vi "Two_neuron_oscillator.vi"() -> ()   [LabVIEW 2016]
uses:
  <vilib>/measure/NI_MABase.lvlib
panel:
  in  "frequency":dbl=0.625 format="%#_13g"
  out "W":T1(graph)
  in  "Modulation":dbl[](array[numeric])=[1.0, 1.0, 1.0, -1.0, 1.0]
  in  "Simulation delay":u32=10
  out "Neurons":T2(graph)
  out "Viewer":T3={"NoPre"=[0, 2, 2], "Pre IDs"=[0, 1, 2, 1, 2], "W"=[1.0, 1.0, 1.0, -1.0, 1.0], "Current"=[1.0, 0.0, 0.0]}
  in  "stop":bool
  in  "Network AER Vectors":T3={"NoPre"=[0, 2, 2], "Pre IDs"=[0, 1, 2, 1, 2], "W"=[1.0, 1.0, 1.0, -1.0, 1.0], "Current"=[1.0, 0.0, 0.0]}
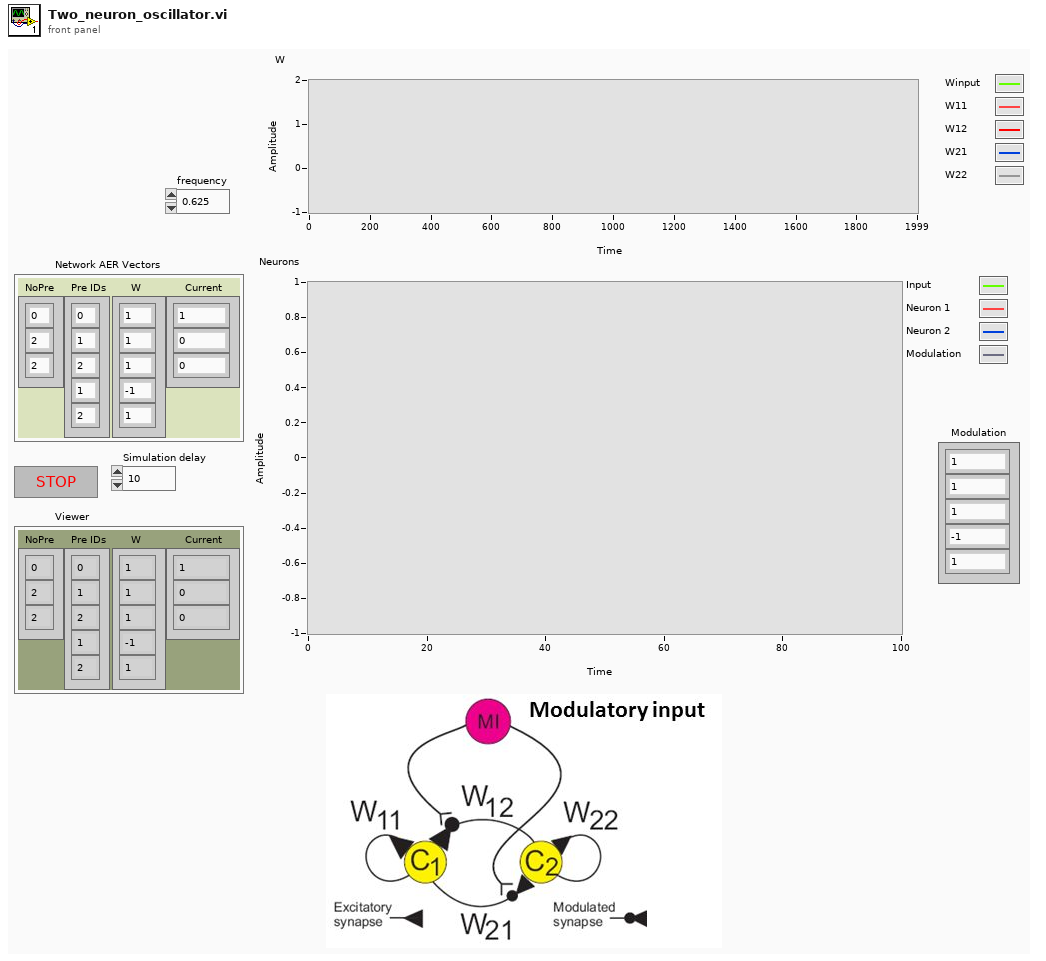
[diagram p1: front panel]
types:
  T1 = cluster{"W[0]":dbl, "W[1]":dbl, "W[2]":dbl, "W[3]":dbl, "W[4]":dbl}
  T2 = cluster{"Current[0]":dbl, "Current[1]":dbl, "Current[2]":dbl, "Current[3]":dbl}
  T3 = cluster{"NoPre":i32[], "Pre IDs":i32[], "W":dbl[], "Current":dbl[]}
  T4 = cluster{"[0]":dbl, "[1]":dbl, "[2]":dbl, "[3]":dbl, "[4]":dbl}
  T5 = cluster{"[0]":dbl, "[1]":dbl, "[2]":dbl, "[3]":dbl}
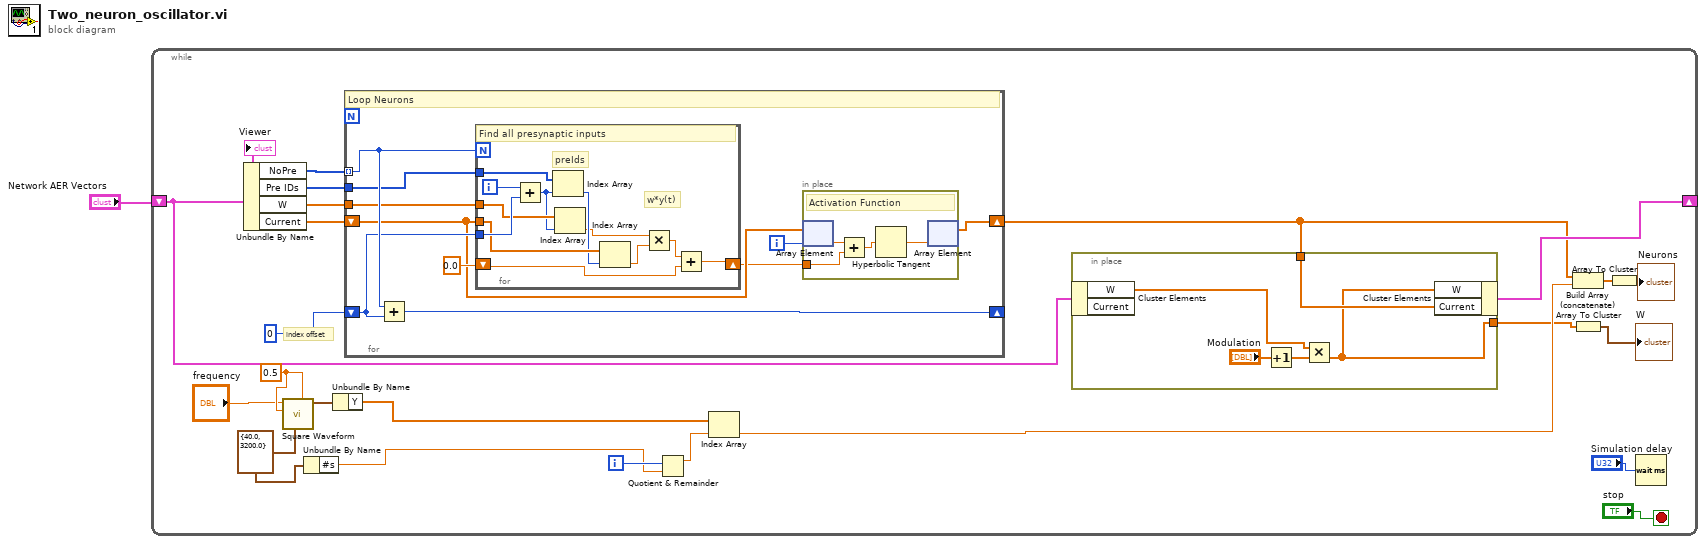
[diagram p0: block diagram]
diagram:
  n1 = while {
    shift-right: [w11] -> _
    shift-left: "Network AER Vectors" -> [w12]
    i -> [w14]
    stop <- "stop" stop-if-true
    w7 = 0.5 ("offset")
    w6 = cluster{"Fs":dbl, "#s":dbl} {"Fs"=40.0, "#s"=3200.0} ("sampling info")
    # "index offset"
    n2 = Unbundle By Name(w12) -> ("NoPre"=w24:i32[], "Pre IDs"=w22:i32[], "W"=w21:dbl[], "Current"=w20:dbl[])
    n3 = call <vilib>:"Square Waveform.vi"("offset"=w7, "sampling info"=w6, "amplitude"=w7, "frequency"="frequency") -> ("signal out"=w5:waveform(dbl))  [unwired: 6 in, 1 out]
    n4 = Unbundle By Name(w6) -> ("#s"=w2:dbl)
    n5 = Unbundle By Name(w5) -> ("Y"=w3:dbl[])
    n6 = for {
      tunnel: w24 -> [w38] mode=indexing
      shift-right: [w39] -> _
      shift-left: 0 -> [w37]
      tunnel: w22 -> [w36]
      tunnel: w21 -> [w30]
      shift-right: [w31] -> w10
      shift-left: w20 -> [w34]
      i -> [w33]
      # "Loop Neurons"
      n7 = Add(x=w38, y=w37) -> (x+y=w39:i32)
      n8 = for {
        N: w38 -> [_]
        tunnel: w37 -> [w54]
        tunnel: w36 -> [w53]
        tunnel: w30 -> [w52]
        tunnel: w34 -> [w51]
        shift-right: [w47] -> w32
        shift-left: 0.0 -> [w45]
        i -> [w55]
        # "w*y(t)"
        # "preIds"
        # "Find all presynaptic inputs"
        n9 = Add(x=w55, y=w54) -> (x+y=w44:i32)
        n10 = Index Array(array=w53, index=w44) -> (element=w50:i32)
        n11 = Index Array(array=w52, index=w44) -> (element=w49:dbl)
        n12 = Index Array(array=w51, index=w50) -> (element=w48:dbl)
        n13 = Multiply(x=w49, y=w48) -> (x*y=w46:dbl)
        n14 = Add(x=w46, y=w45) -> (x+y=w47:dbl)
      }
      n15 = in-place {
        in-place-border: w32 -> [w43]
        # "Activation Function"
        n16 = in-place-array #1(w34, w33) -> (w41:dbl)
        n17 = Add(x=w41, y=w43) -> (x+y=w40:dbl)
        n18 = Hyperbolic Tangent(1:w40) -> (0:w42:dbl)
        n19 = in-place-array #1(w42) -> (w31:dbl[])  [unwired: 1 out]
      }
    }
    n20 = Quotient & Remainder(x=w14, y=w2) -> (x-y*floor(x/y)=w15:dbl)  [unwired: 1 out]
    n21 = Index Array(array=w3, index=w15) -> (element=w13:dbl)
    n22 = in-place {
      in-place-border: w10 -> [w29]
      in-place-border: [w26] -> w9
      n23 = in-place-cluster #2(w12) -> ("W"=w25:dbl[])  [unwired: 1 out]
      n24 = Increment(x="Modulation") -> (x+1=w28:dbl[])
      n25 = Multiply(x=w25, y=w28) -> (x*y=w26:dbl[])
      n26 = in-place-cluster #2("W"=w26, "Current"=w29) -> (w11:T3)
    }
    n27 = Build Array (concatenate)(w10, w13) -> (w16:dbl[])
    n28 = Array To Cluster(array=w9) -> (cluster=→"W":T4)
    n29 = Array To Cluster(array=w16) -> (cluster=→"Neurons":T5)
    n30 = Wait (ms)(milliseconds to wait="Simulation delay") -> ()  [unwired: 1 out]
    "Viewer" <- w12
  }
